vi "Alt 2 Num.vi"(3 "Alt Ctl":T1 {"Alt Digit 100" min=0 max=9 step=1; "Alt Digit 100" min=0 max=9 step=1; "Alt Digit 100" min=0 max=9 step=1; "Alt Digit 100" min=0 max=9 step=1; "Alt Digit 100" min=0 max=9 step=1}) -> (1 "Alt":i32)   [LabVIEW 2013]
uses:
  Type Defs/Alt Control.ctl
  Type Defs/Alt Digit 100 New.ctl
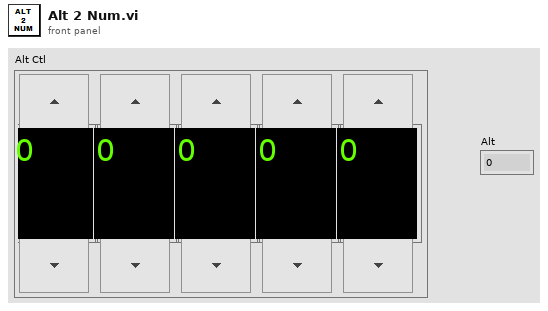
[diagram p1: front panel]
types:
  T1 = typedef "Alt Control.ctl" = cluster{"Alt Digit 100":T2, "Alt Digit 100":T2, "Alt Digit 100":T2, "Alt Digit 100":T2, "Alt Digit 100":T2}
  T2 = typedef "Alt Digit 100 New.ctl" = i8
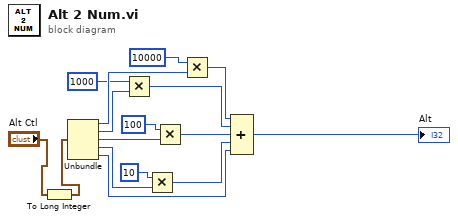
[diagram p0: block diagram]
diagram:
  n1 = To Long Integer(number="Alt Ctl") -> (32bit integer=w1:cluster{i32, i32, i32, i32, i32})
  n2 = Unbundle(w1) -> (w16:i32, w11:i32, w10:i32, w9:i32, w4:i32)
  n3 = Multiply(x=1000, y=w11) -> (x*y=w7:i32)
  n4 = Multiply(x=10, y=w9) -> (x*y=w5:i32)
  n5 = Multiply(x=100, y=w10) -> (x*y=w6:i32)
  n6 = Multiply(x=10000, y=w16) -> (x*y=w8:i32)
  n7 = Compound Arithmetic op=ADD(w8, w7, w6, w5, w4) -> (→"Alt":i32)
